vi "PhotonTrackedTarget_CreateFromPacket.vi"(9 "StartByte":i32, 11 "RawData":u8[](array[numeric])) -> (1 "NextByte":i32, 3 "TrackedTarget":T1={"Yaw"=0.0, "Pitch"=0.0, "Area"=0.0, "Skew"=0.0, "TargetCorners"=[], "Pose"={"TRANSLATION"={"X"=0.0, "Y"=0.0}, "ROTATION"={"VALUE"=0.0, "COS"=1.0, "SIN"=0.0}}} {"Pose"."ROTATION"."SIN" format="%13.4f"; "Pose"."ROTATION"."COS" format="%13.4f"; "Pose"."ROTATION"."VALUE" format="%13.4f"; "Pose"."TRANSLATION"."Y" format="%14.3f"; "Pose"."TRANSLATION"."X" format="%14.3f"})   [LabVIEW 2019, in "PhotonVisionLib.lvlib"]
doc: "Internal function to parse the data for each target returned by PhotonCamera_GetLatestResult.\n\nInputs:\n - RawData -- Byte array containing the data to parse.\n\nOutputs:\n - TrackedTarget -- Parsed TrackedTarget cluster."
uses:
  PhotonVisionLib.lvlib
  TypeDef/PhotonTrackedTargetType.ctl
  TypeDef/TargetCornerType.ctl
  <vilib>/Rock Robotics/WPI/ThirdParty/JAS_Junk/TrajLib/POSE2D.ctl
  <vilib>/Rock Robotics/WPI/ThirdParty/JAS_Junk/TrajLib/TRANSLATION2D.ctl
  <vilib>/Rock Robotics/WPI/ThirdParty/JAS_Junk/TrajLib/ROTATION2D.ctl
  <vilib>/Rock Robotics/WPI/ThirdParty/JAS_Junk/TrajLib/Rotation_CreateAngle.vi
  <vilib>/Rock Robotics/WPI/ThirdParty/JAS_Junk/TrajLib/Translation_Create.vi
  <vilib>/Rock Robotics/WPI/ThirdParty/JAS_Junk/TrajLib/Trajectory_Library.lvlib
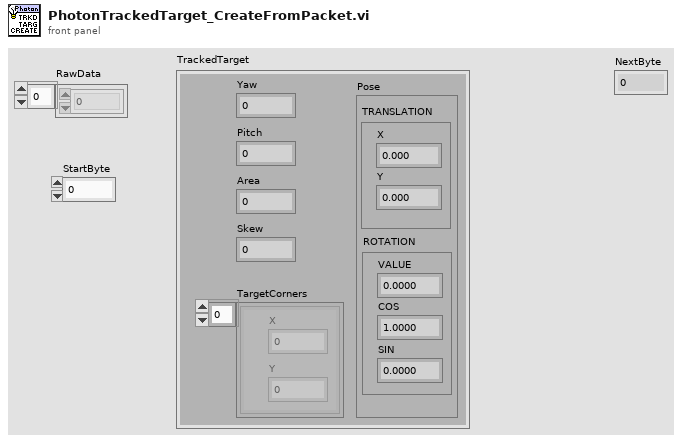
[diagram p1: front panel]
types:
  T1 = typedef "PhotonVisionLib.lvlib/PhotonTrackedTargetType.ctl" = cluster{"Yaw":dbl, "Pitch":dbl, "Area":dbl, "Skew":dbl, "TargetCorners":T2[], "Pose":T3}
  T2 = typedef "PhotonVisionLib.lvlib/TargetCornerType.ctl" = cluster{"X":dbl, "Y":dbl}
  T3 = typedef "Trajectory_Library.lvlib/POSE2D.ctl" = cluster{"TRANSLATION":T4, "ROTATION":T5}
  T4 = typedef "Trajectory_Library.lvlib/TRANSLATION2D.ctl" = cluster{"X":dbl, "Y":dbl}
  T5 = typedef "Trajectory_Library.lvlib/ROTATION2D.ctl" = cluster{"VALUE":dbl, "COS":dbl, "SIN":dbl}
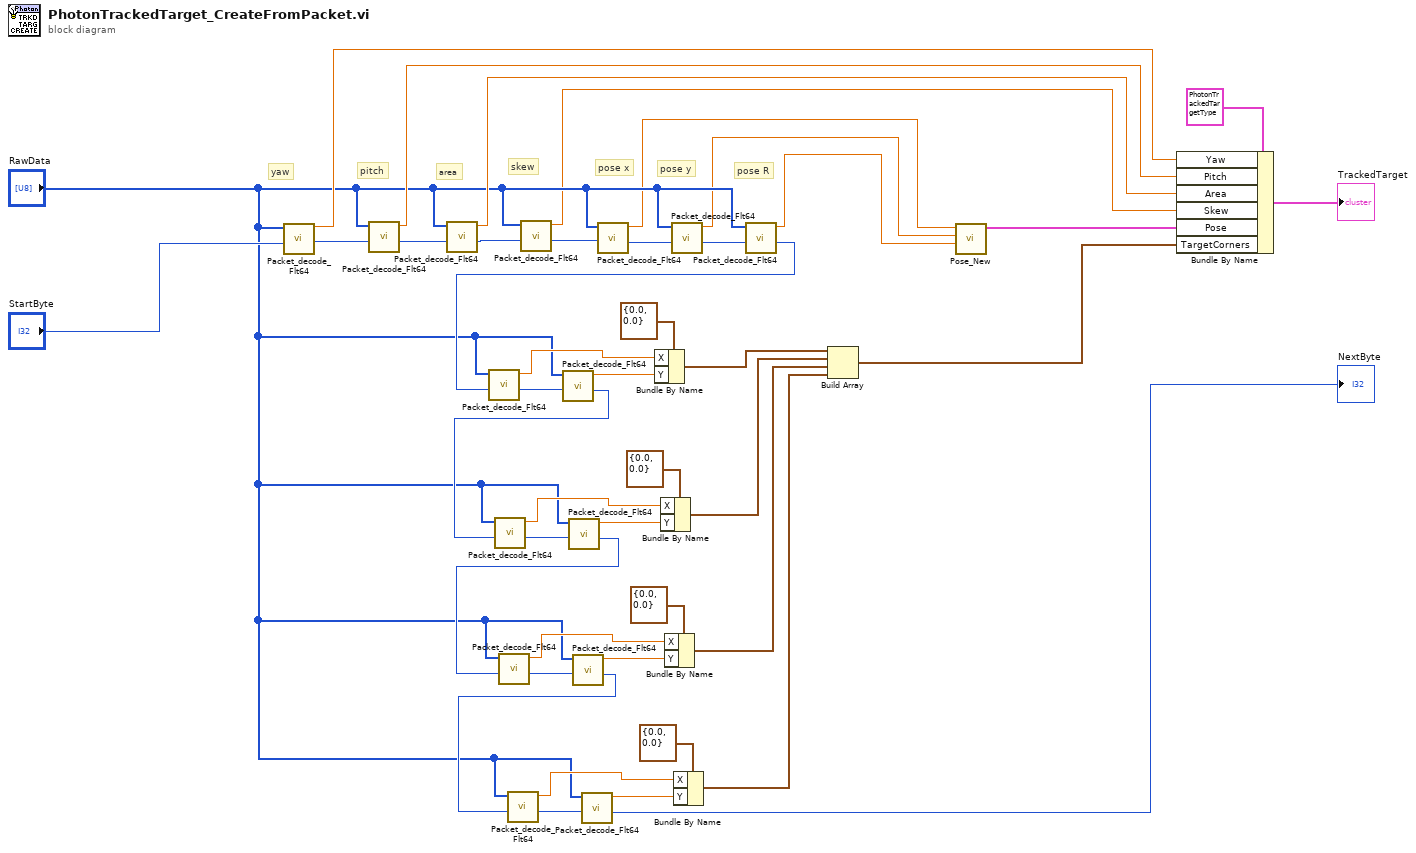
[diagram p0: block diagram]
diagram:
  # "pose R"
  # "pose y"
  # "pose x"
  # "skew"
  # "area"
  # "pitch"
  # "yaw"
  n1 = call "Packet_decode_Flt64.vi"("StartByte"="StartByte", "RawData"="RawData") -> ("NextByte"=w41:i32, "Flt64_Value"=w44:dbl)  [unwired: 8 in]
  n2 = call "Packet_decode_Flt64.vi"("StartByte"=w41, "RawData"="RawData") -> ("NextByte"=w39:i32, "Flt64_Value"=w40:dbl)  [unwired: 8 in]
  n3 = call "Packet_decode_Flt64.vi"("StartByte"=w39, "RawData"="RawData") -> ("NextByte"=w8:i32, "Flt64_Value"=w15:dbl)  [unwired: 8 in]
  n4 = call "Packet_decode_Flt64.vi"("StartByte"=w8, "RawData"="RawData") -> ("NextByte"=w7:i32, "Flt64_Value"=w5:dbl)  [unwired: 8 in]
  n5 = call "Packet_decode_Flt64.vi"("StartByte"=w7, "RawData"="RawData") -> ("NextByte"=w38:i32, "Flt64_Value"=w4:dbl)  [unwired: 8 in]
  n6 = call "Packet_decode_Flt64.vi"("StartByte"=w38, "RawData"="RawData") -> ("NextByte"=w37:i32, "Flt64_Value"=w3:dbl)  [unwired: 8 in]
  n7 = call "Packet_decode_Flt64.vi"("StartByte"=w37, "RawData"="RawData") -> ("NextByte"=w14:i32, "Flt64_Value"=w2:dbl)  [unwired: 8 in]
  n8 = call "Packet_decode_Flt64.vi"("StartByte"=w14, "RawData"="RawData") -> ("NextByte"=w36:i32, "Flt64_Value"=w33:dbl)  [unwired: 8 in]
  n9 = call "Packet_decode_Flt64.vi"("StartByte"=w36, "RawData"="RawData") -> ("NextByte"=w13:i32, "Flt64_Value"=w34:dbl)  [unwired: 8 in]
  n10 = call "Packet_decode_Flt64.vi"("StartByte"=w13, "RawData"="RawData") -> ("NextByte"=w32:i32, "Flt64_Value"=w29:dbl)  [unwired: 8 in]
  n11 = call "Packet_decode_Flt64.vi"("StartByte"=w32, "RawData"="RawData") -> ("NextByte"=w12:i32, "Flt64_Value"=w30:dbl)  [unwired: 8 in]
  n12 = call "Packet_decode_Flt64.vi"("StartByte"=w12, "RawData"="RawData") -> ("NextByte"=w28:i32, "Flt64_Value"=w25:dbl)  [unwired: 8 in]
  n13 = call "Packet_decode_Flt64.vi"("StartByte"=w28, "RawData"="RawData") -> ("NextByte"=w11:i32, "Flt64_Value"=w26:dbl)  [unwired: 8 in]
  n14 = call "Packet_decode_Flt64.vi"("StartByte"=w11, "RawData"="RawData") -> ("NextByte"=w24:i32, "Flt64_Value"=w21:dbl)  [unwired: 8 in]
  n15 = call "Packet_decode_Flt64.vi"("StartByte"=w24, "RawData"="RawData") -> ("NextByte"=→"NextByte":i32, "Flt64_Value"=w22:dbl)  [unwired: 8 in]
  n16 = Bundle By Name(cluster=T2 {"X"=0.0, "Y"=0.0} ("TargetCorner"), "X"=w33, "Y"=w34) -> (w20:T2)
  n17 = Bundle By Name(cluster=T2 {"X"=0.0, "Y"=0.0} ("TargetCorner"), "X"=w29, "Y"=w30) -> (w19:T2)
  n18 = Bundle By Name(cluster=T2 {"X"=0.0, "Y"=0.0} ("TargetCorner"), "X"=w25, "Y"=w26) -> (w18:T2)
  n19 = Bundle By Name(cluster=T2 {"X"=0.0, "Y"=0.0} ("TargetCorner"), "X"=w21, "Y"=w22) -> (w17:T2)
  n20 = Build Array(w20, w19, w18, w17) -> (w16:T2[])
  n21 = call <vilib>:"Pose_New.vi"("Heading"=w2, "Y"=w3, "X"=w4) -> ("out POSe"=w1:T3)  [unwired: 8 in]
  n22 = Bundle By Name(cluster=T1 {"Yaw"=0.0, "Pitch"=0.0, "Area"=0.0, "Skew"=0.0, "TargetCorners"=[], "Pose"={"TRANSLATION"={"X"=0.0, "Y"=0.0}, "ROTATION"={"VALUE"=0.0, "COS"=1.0, "SIN"=0.0}}} ("PhotonTrackedTarget"), "Yaw"=w44, "Pitch"=w40, "Area"=w15, "Skew"=w5, "Pose"=w1, "TargetCorners"=w16) -> (→"TrackedTarget":T1)
